vi "Read volume table.vi"(8 "error in (no error)":errorcluster, 10 "File path":path, 11 "Tomo in":refnum<class "Tomo.lvclass">) -> (0 "error out":errorcluster, 2 "System Array":dbl[][](array[numeric]), 3 "Tomo out":refnum<class "Tomo.lvclass">)   [LabVIEW 2012, in "Tomo.lvclass"]
uses:
  Tomo.lvclass
  <vilib>/Utility/file.llb/Read From Spreadsheet File (DBL).vi
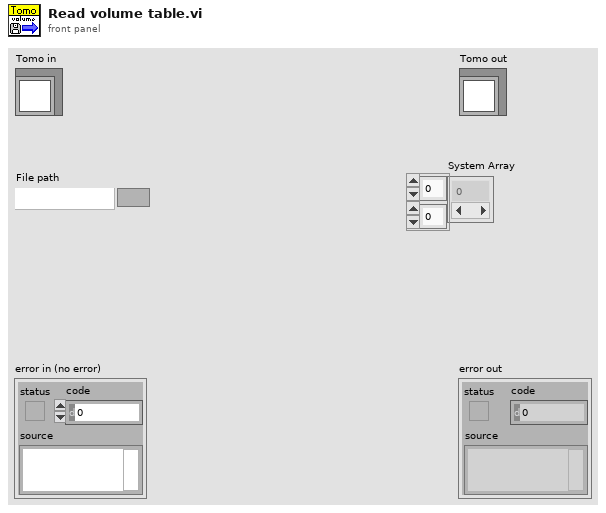
[diagram p1: front panel]
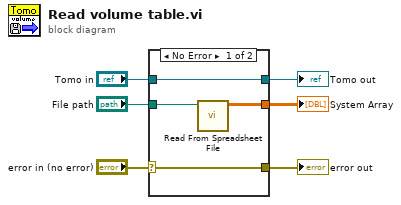
[diagram p0: block diagram]
diagram:
  n1 = case shown="No Error" "error in (no error)" {
    selector: "error in (no error)" -> [w9 w12]
    tunnel: [w9 w12] -> w5
    tunnel: [w10 w11] -> w3
    tunnel: "Tomo in" -> [w10 w11]
    tunnel: "File path" -> [w8 _]
    tunnel: [w7 _] -> w1
    frame No Error {
      n2 = call-poly <vilib>:"Read From Spreadsheet File.vi"("file path (dialog if empty)"=w8) -> ("all rows"=w7:dbl[][])  [unwired: 6 in, 4 out]
    }
    frame Error {
    }
  }
  "error out" <- w5
  "Tomo out" <- w3
  "System Array" <- w1
